vi "VAM-A-archive.vi"(1 "VAM-A":T2 {"63 B_NI6220" format="%.4g"; "62" format="%.4g"; "61" format="%.4g"; "60" format="%.4g"; "59" format="%.4g"; "58" format="%.4g"; "57" format="%.4g"; "56" format="%.4g"; "55" format="%.4g"; "54" format="%.4g"; "53" format="%.4g"; "52" format="%.4g"; "51" format="%.4g"; "50" format="%.4g"; "49" format="%.4g"; "48" format="%.4g"; "47" format="%.4g"; "46" format="%.4g"; "45" format="%.4g"; "44" format="%.4g"; "43" format="%.4g"; "42" format="%.4g"; "41" format="%.4g"; "40" format="%.4g"; "39 WCM2DMin" format="%.4g"; "38 WCM2GMin" format="%.4g"; "37 WCM2BMin" format="%.4g"; "36 WCM2HMin" format="%.4g"; "35 WCM2DMax" format="%.4g"; "34 WCM2GMax" format="%.4g"; "33 WCM2BMax" format="%.4g"; "32 WCM2HMax" format="%.4g"; "31" format="%.4g"; "30" format="%.4g"; "29" format="%.4g"; "28" format="%.4g"; "27" format="%.4g"; "26" format="%.4g"; "25" format="%.4g"; "24" format="%.4g"; "23" format="%.4g"; "22" format="%.4g"; "21" format="%.4g"; "20 ACQ Vide TPG300 PIQ63" format="%.4g"; "19 ACQ Libre" format="%.5g"; "18 ACQ Libre" format="%.5g"; "17 ACQ Vide Ecran PIQ53/63" format="%.5g"; "16 ACQ Vide Dip PIQ27/33" format="%.5g"; "15 ACQ Vide Miroir PIQ21" format="%.5g"; "14 ACQ Vide Section PIQ16" format="%.5g"; "13 ACQ Vide Canon PIQ12" format="%.5g"; "12 ACQ Vide PI Guide HF" format="%.5f"; "11 ACQ Vide Chambre" format="%.4g"; "10 ACQ Vide Section" format="%.4g"; "09" format="%.4g"; "08" format="%.4g"; "07" format="%.4g"; "06" format="%.4g"; "05" format="%.4g"; "04" format="%.4g"; "03" format="%.4g"; "02 ACQ Evénement" format="%.4g"; "01 ACQ Variables" format="%.4g"; "00 ACQ Auxiliare" format="%.4g"}, 2 "C5_IN_DIO96":T1, 3 "archive in":T3={"sync"={"elyse/sync/NI6071E/delay"=1.5500000000000005, "elyse/sync/NI6071E/width"=1.0, "elyse/sync/frequency/delay"=10.0, "elyse/sync/frequency/width"=181000.0, "elyse/sync/WCM/delay"=2177.9, "elyse/sync/WCM/width"=10.0, "elyse/sync/modulator/delay"=2182.400000000002, "elyse/sync/modulator/width"=3.0, "elyse/sync/HF/delay"=2175.0, "elyse/sync/HF/width"=3.0, "elyse/sync/Faraday/delay"=5080.0, "elyse/sync/Faraday/width"=100.0, "elyse/sync/Oscilloscope/delay"=2175.0, "elyse/sync/Oscilloscope/width"=2.8, "elyse/sync/50Hz_20MHz/delay"=1.0, "elyse/sync/50Hz_20MHz/width"=5000.0, "elyse/sync/laser_HF/delay"=0.35, "elyse/sync/laser_HF/width"=0.35, "elyse/sync/IMAC/delay"=2176.0, "elyse/sync/IMAC/width"=100.0, "elyse/sync/laser/delay"=2008.3, "elyse/sync/laser/width"=10.0, "elyse/sync/oscilloscope1/delay"=2175.0, "elyse/sync/oscilloscope1/width"=10.0, "elyse/sync/oscilloscope2/delay"=2175.0, "elyse/sync/oscilloscope2/width"=100.0, "elyse/sync/detection1/delay"=500.0, "elyse/sync/detection1/width"=500.0, "elyse/sync/detection1/delay"=0.3, "elyse/sync/detection2/width"=10.0, "elyse/sync/machine/delay"=2175.0, "elyse/sync/machine/width"=100.0, "elyse/sync/n_selection"=4.0}, "HT"={"elyse/HT/voltage/set_value"=6.5, "elyse/HT/voltage/value"=1.5625e-08, "elyse/HT/current/value"=0.0, "elyse/preamplifier/set_value"=1.5625e-08, "elyse/preamplifier/value"=0.0}, "HF"={"elyse/HF/attenuator/value"=-0.01903046052094623, "elyse/HF/dephaser/value"=-18.585806237727724, "elyse/HF/dephaser/value_manuel"=-78.82860725035081, "elyse/HF/canon/value"=0.0, "elyse/HF/section/value"=-18.585806237727724}, "vacuum"={"elyse/vacuum/preparation_chamber/state"=TRUE, "elyse/vacuum/preparation_chamber/measurement"=0.0, "elyse/vacuum/HF/state"=TRUE, "elyse/vacuum/HF/measurement"=0.0, "elyse/vacuum/canon/state"=TRUE, "elyse/vacuum/canon/measurement"=0.0, "elyse/vacuum/section/state"=TRUE, "elyse/vacuum/section/measurement"=0.0, "elyse/vacuum/dipole1/state"=TRUE, "elyse/vacuum/dipole1/measurement"=0.0, "elyse/vacuum/screen1/state"=TRUE, "elyse/vacuum/screen1/measurement"=0.0, "elyse/vacuum/mirror/state"=TRUE, "elyse/vacuum/mirror/measurement"=0.0, "elyse/vacuum/tpg300_section/state"=TRUE, "elyse/vacuum/tpg300_section/measurement"=0.0, "elyse/vacuum/valves/cathode/state"=FALSE, "elyse/vacuum/valves/injection/state"=FALSE}, "modulator"={"elyse/modulator/focale1/current/value"=0.0, "elyse/modulator/focale2/current/value"=0.0, "elyse/modulator/focale3/current/value"=0.0, "elyse/modulator/LAR/voltage/value"=0.0, "elyse/modulator/line_end/current/value"=0.0, "elyse/modulator/thyratron/currents/power/value"=0.0, "elyse/modulator/thyratron_reservoir/current/value"=0.0, "elyse/modulator/paramagnetization/current/value"=0.0, "elyse/modulator/thyratron/voltages/heating/value"=0.0, "elyse/modulator/thyratron/currents/heating/value"=0.0, "elyse/modulator/klystron/currents/power/value"=0.0, "elyse/modulator/klystron/voltages/power/value"=0.0, "elyse/modulator/klystron/currents/heating/value"=0.0, "elyse/modulator/klystron/voltages/heating/value"=0.0}, "cooling"={"elyse/cooling/section/temperature/set_value"=28.0, "elyse/cooling/section/temperature/measurement"=27.96142578125, "elyse/cooling/canon/temperature/set_value"=20.2, "elyse/cooling/canon/temperature/measurement"=26.69921875}, "magnets"={"elyse/magnets/focale/set_value"=0.0, "elyse/magnets/focale/value"=0.0, "elyse/magnets/phase_HF_laser/set_value"=0.0, "elyse/magnets/phase_HF_laser/value"=0.0, "elyse/magnets/dipole1/set_value"=0.0, "elyse/magnets/dipole1/value"=0.0, "elyse/magnets/dipole2/set_value"=0.0, "elyse/magnets/dipole2/value"=0.0, "elyse/magnets/Cor_H1/set_value"=0.0, "elyse/magnets/Cor_H1/value"=0.0, "elyse/magnets/Cor_V1/set_value"=0.0, "elyse/magnets/Cor_V1/value"=0.0, "elyse/magnets/Cor_H2/set_value"=0.0, "elyse/magnets/Cor_H2/value"=0.0, "elyse/magnets/Cor_V2/set_value"=0.0, "elyse/magnets/Cor_V2/value"=0.0, "elyse/magnets/Cor_H3/set_value"=0.0, "elyse/magnets/Cor_H3/value"=0.0, "elyse/magnets/Cor_V3/set_value"=-5.0, "elyse/magnets/Cor_V3/value"=0.0, "elyse/magnets/Cor_H4/set_value"=0.0, "elyse/magnets/Cor_H4/value"=0.0, "elyse/magnets/Cor_V4/set_value"=0.0, "elyse/magnets/Cor_V4/value"=0.0, "elyse/magnets/Cor_H5/set_value"=0.0, "elyse/magnets/Cor_H5/value"=0.0, "elyse/magnets/Cor_V5/set_value"=0.0, "elyse/magnets/Cor_V5/value"=0.0, "elyse/magnets/triplet1-1/set_value"=0.0, "elyse/magnets/triplet1-1/value"=0.0, "elyse/magnets/triplet1-2/set_value"=0.0, "elyse/magnets/triplet1-2/value"=0.0, "elyse/magnets/triplet2-1/set_value"=0.0, "elyse/magnets/triplet2-1/value"=0.0, "elyse/magnets/triplet2-2/set_value"=0.0, "elyse/magnets/triplet2-2/value"=0.0, "elyse/magnets/qudrupole1/set_value"=0.0, "elyse/magnets/qudrupole1/value"=0.0, "elyse/magnets/qudrupole2/set_value"=0.0, "elyse/magnets/qudrupole2/value"=0.0}, "time"={"elyse/timestamp"=0.0}}) -> (0 "archive out":T3={"sync"={"elyse/sync/NI6071E/delay"=1.5500000000000005, "elyse/sync/NI6071E/width"=1.0, "elyse/sync/frequency/delay"=10.0, "elyse/sync/frequency/width"=181000.0, "elyse/sync/WCM/delay"=2177.9, "elyse/sync/WCM/width"=10.0, "elyse/sync/modulator/delay"=2182.400000000002, "elyse/sync/modulator/width"=3.0, "elyse/sync/HF/delay"=2175.0, "elyse/sync/HF/width"=3.0, "elyse/sync/Faraday/delay"=5080.0, "elyse/sync/Faraday/width"=100.0, "elyse/sync/Oscilloscope/delay"=2175.0, "elyse/sync/Oscilloscope/width"=2.8, "elyse/sync/50Hz_20MHz/delay"=1.0, "elyse/sync/50Hz_20MHz/width"=5000.0, "elyse/sync/laser_HF/delay"=0.35, "elyse/sync/laser_HF/width"=0.35, "elyse/sync/IMAC/delay"=2176.0, "elyse/sync/IMAC/width"=100.0, "elyse/sync/laser/delay"=2008.3, "elyse/sync/laser/width"=10.0, "elyse/sync/oscilloscope1/delay"=2175.0, "elyse/sync/oscilloscope1/width"=10.0, "elyse/sync/oscilloscope2/delay"=2175.0, "elyse/sync/oscilloscope2/width"=100.0, "elyse/sync/detection1/delay"=500.0, "elyse/sync/detection1/width"=500.0, "elyse/sync/detection1/delay"=0.3, "elyse/sync/detection2/width"=10.0, "elyse/sync/machine/delay"=2175.0, "elyse/sync/machine/width"=100.0, "elyse/sync/n_selection"=4.0}, "HT"={"elyse/HT/voltage/set_value"=6.5, "elyse/HT/voltage/value"=1.5625e-08, "elyse/HT/current/value"=0.0, "elyse/preamplifier/set_value"=1.5625e-08, "elyse/preamplifier/value"=0.0}, "HF"={"elyse/HF/attenuator/value"=-0.01903046052094623, "elyse/HF/dephaser/value"=-18.585806237727724, "elyse/HF/dephaser/value_manuel"=-78.82860725035081, "elyse/HF/canon/value"=0.0, "elyse/HF/section/value"=-18.585806237727724}, "vacuum"={"elyse/vacuum/preparation_chamber/state"=TRUE, "elyse/vacuum/preparation_chamber/measurement"=0.0, "elyse/vacuum/HF/state"=TRUE, "elyse/vacuum/HF/measurement"=0.0, "elyse/vacuum/canon/state"=TRUE, "elyse/vacuum/canon/measurement"=0.0, "elyse/vacuum/section/state"=TRUE, "elyse/vacuum/section/measurement"=0.0, "elyse/vacuum/dipole1/state"=TRUE, "elyse/vacuum/dipole1/measurement"=0.0, "elyse/vacuum/screen1/state"=TRUE, "elyse/vacuum/screen1/measurement"=0.0, "elyse/vacuum/mirror/state"=TRUE, "elyse/vacuum/mirror/measurement"=0.0, "elyse/vacuum/tpg300_section/state"=TRUE, "elyse/vacuum/tpg300_section/measurement"=0.0, "elyse/vacuum/valves/cathode/state"=FALSE, "elyse/vacuum/valves/injection/state"=FALSE}, "modulator"={"elyse/modulator/focale1/current/value"=0.0, "elyse/modulator/focale2/current/value"=0.0, "elyse/modulator/focale3/current/value"=0.0, "elyse/modulator/LAR/voltage/value"=0.0, "elyse/modulator/line_end/current/value"=0.0, "elyse/modulator/thyratron/currents/power/value"=0.0, "elyse/modulator/thyratron_reservoir/current/value"=0.0, "elyse/modulator/paramagnetization/current/value"=0.0, "elyse/modulator/thyratron/voltages/heating/value"=0.0, "elyse/modulator/thyratron/currents/heating/value"=0.0, "elyse/modulator/klystron/currents/power/value"=0.0, "elyse/modulator/klystron/voltages/power/value"=0.0, "elyse/modulator/klystron/currents/heating/value"=0.0, "elyse/modulator/klystron/voltages/heating/value"=0.0}, "cooling"={"elyse/cooling/section/temperature/set_value"=28.0, "elyse/cooling/section/temperature/measurement"=27.96142578125, "elyse/cooling/canon/temperature/set_value"=20.2, "elyse/cooling/canon/temperature/measurement"=26.69921875}, "magnets"={"elyse/magnets/focale/set_value"=0.0, "elyse/magnets/focale/value"=0.0, "elyse/magnets/phase_HF_laser/set_value"=0.0, "elyse/magnets/phase_HF_laser/value"=0.0, "elyse/magnets/dipole1/set_value"=0.0, "elyse/magnets/dipole1/value"=0.0, "elyse/magnets/dipole2/set_value"=0.0, "elyse/magnets/dipole2/value"=0.0, "elyse/magnets/Cor_H1/set_value"=0.0, "elyse/magnets/Cor_H1/value"=0.0, "elyse/magnets/Cor_V1/set_value"=0.0, "elyse/magnets/Cor_V1/value"=0.0, "elyse/magnets/Cor_H2/set_value"=0.0, "elyse/magnets/Cor_H2/value"=0.0, "elyse/magnets/Cor_V2/set_value"=0.0, "elyse/magnets/Cor_V2/value"=0.0, "elyse/magnets/Cor_H3/set_value"=0.0, "elyse/magnets/Cor_H3/value"=0.0, "elyse/magnets/Cor_V3/set_value"=-5.0, "elyse/magnets/Cor_V3/value"=0.0, "elyse/magnets/Cor_H4/set_value"=0.0, "elyse/magnets/Cor_H4/value"=0.0, "elyse/magnets/Cor_V4/set_value"=0.0, "elyse/magnets/Cor_V4/value"=0.0, "elyse/magnets/Cor_H5/set_value"=0.0, "elyse/magnets/Cor_H5/value"=0.0, "elyse/magnets/Cor_V5/set_value"=0.0, "elyse/magnets/Cor_V5/value"=0.0, "elyse/magnets/triplet1-1/set_value"=0.0, "elyse/magnets/triplet1-1/value"=0.0, "elyse/magnets/triplet1-2/set_value"=0.0, "elyse/magnets/triplet1-2/value"=0.0, "elyse/magnets/triplet2-1/set_value"=0.0, "elyse/magnets/triplet2-1/value"=0.0, "elyse/magnets/triplet2-2/set_value"=0.0, "elyse/magnets/triplet2-2/value"=0.0, "elyse/magnets/qudrupole1/set_value"=0.0, "elyse/magnets/qudrupole1/value"=0.0, "elyse/magnets/qudrupole2/set_value"=0.0, "elyse/magnets/qudrupole2/value"=0.0}, "time"={"elyse/timestamp"=0.0}})   [LabVIEW 2020]
uses:
  archive.ctl
  sync_type_def.ctl
  HT_type-def.ctl
  HF_type_def.ctl
  vacuum_type_def.ctl
  modulator_type_def.ctl
  water_cooling_type_def.ctl
  all_magnets_type_def.ctl
  <vilib>/ptbypt/NI_PtbyPt.lvlib
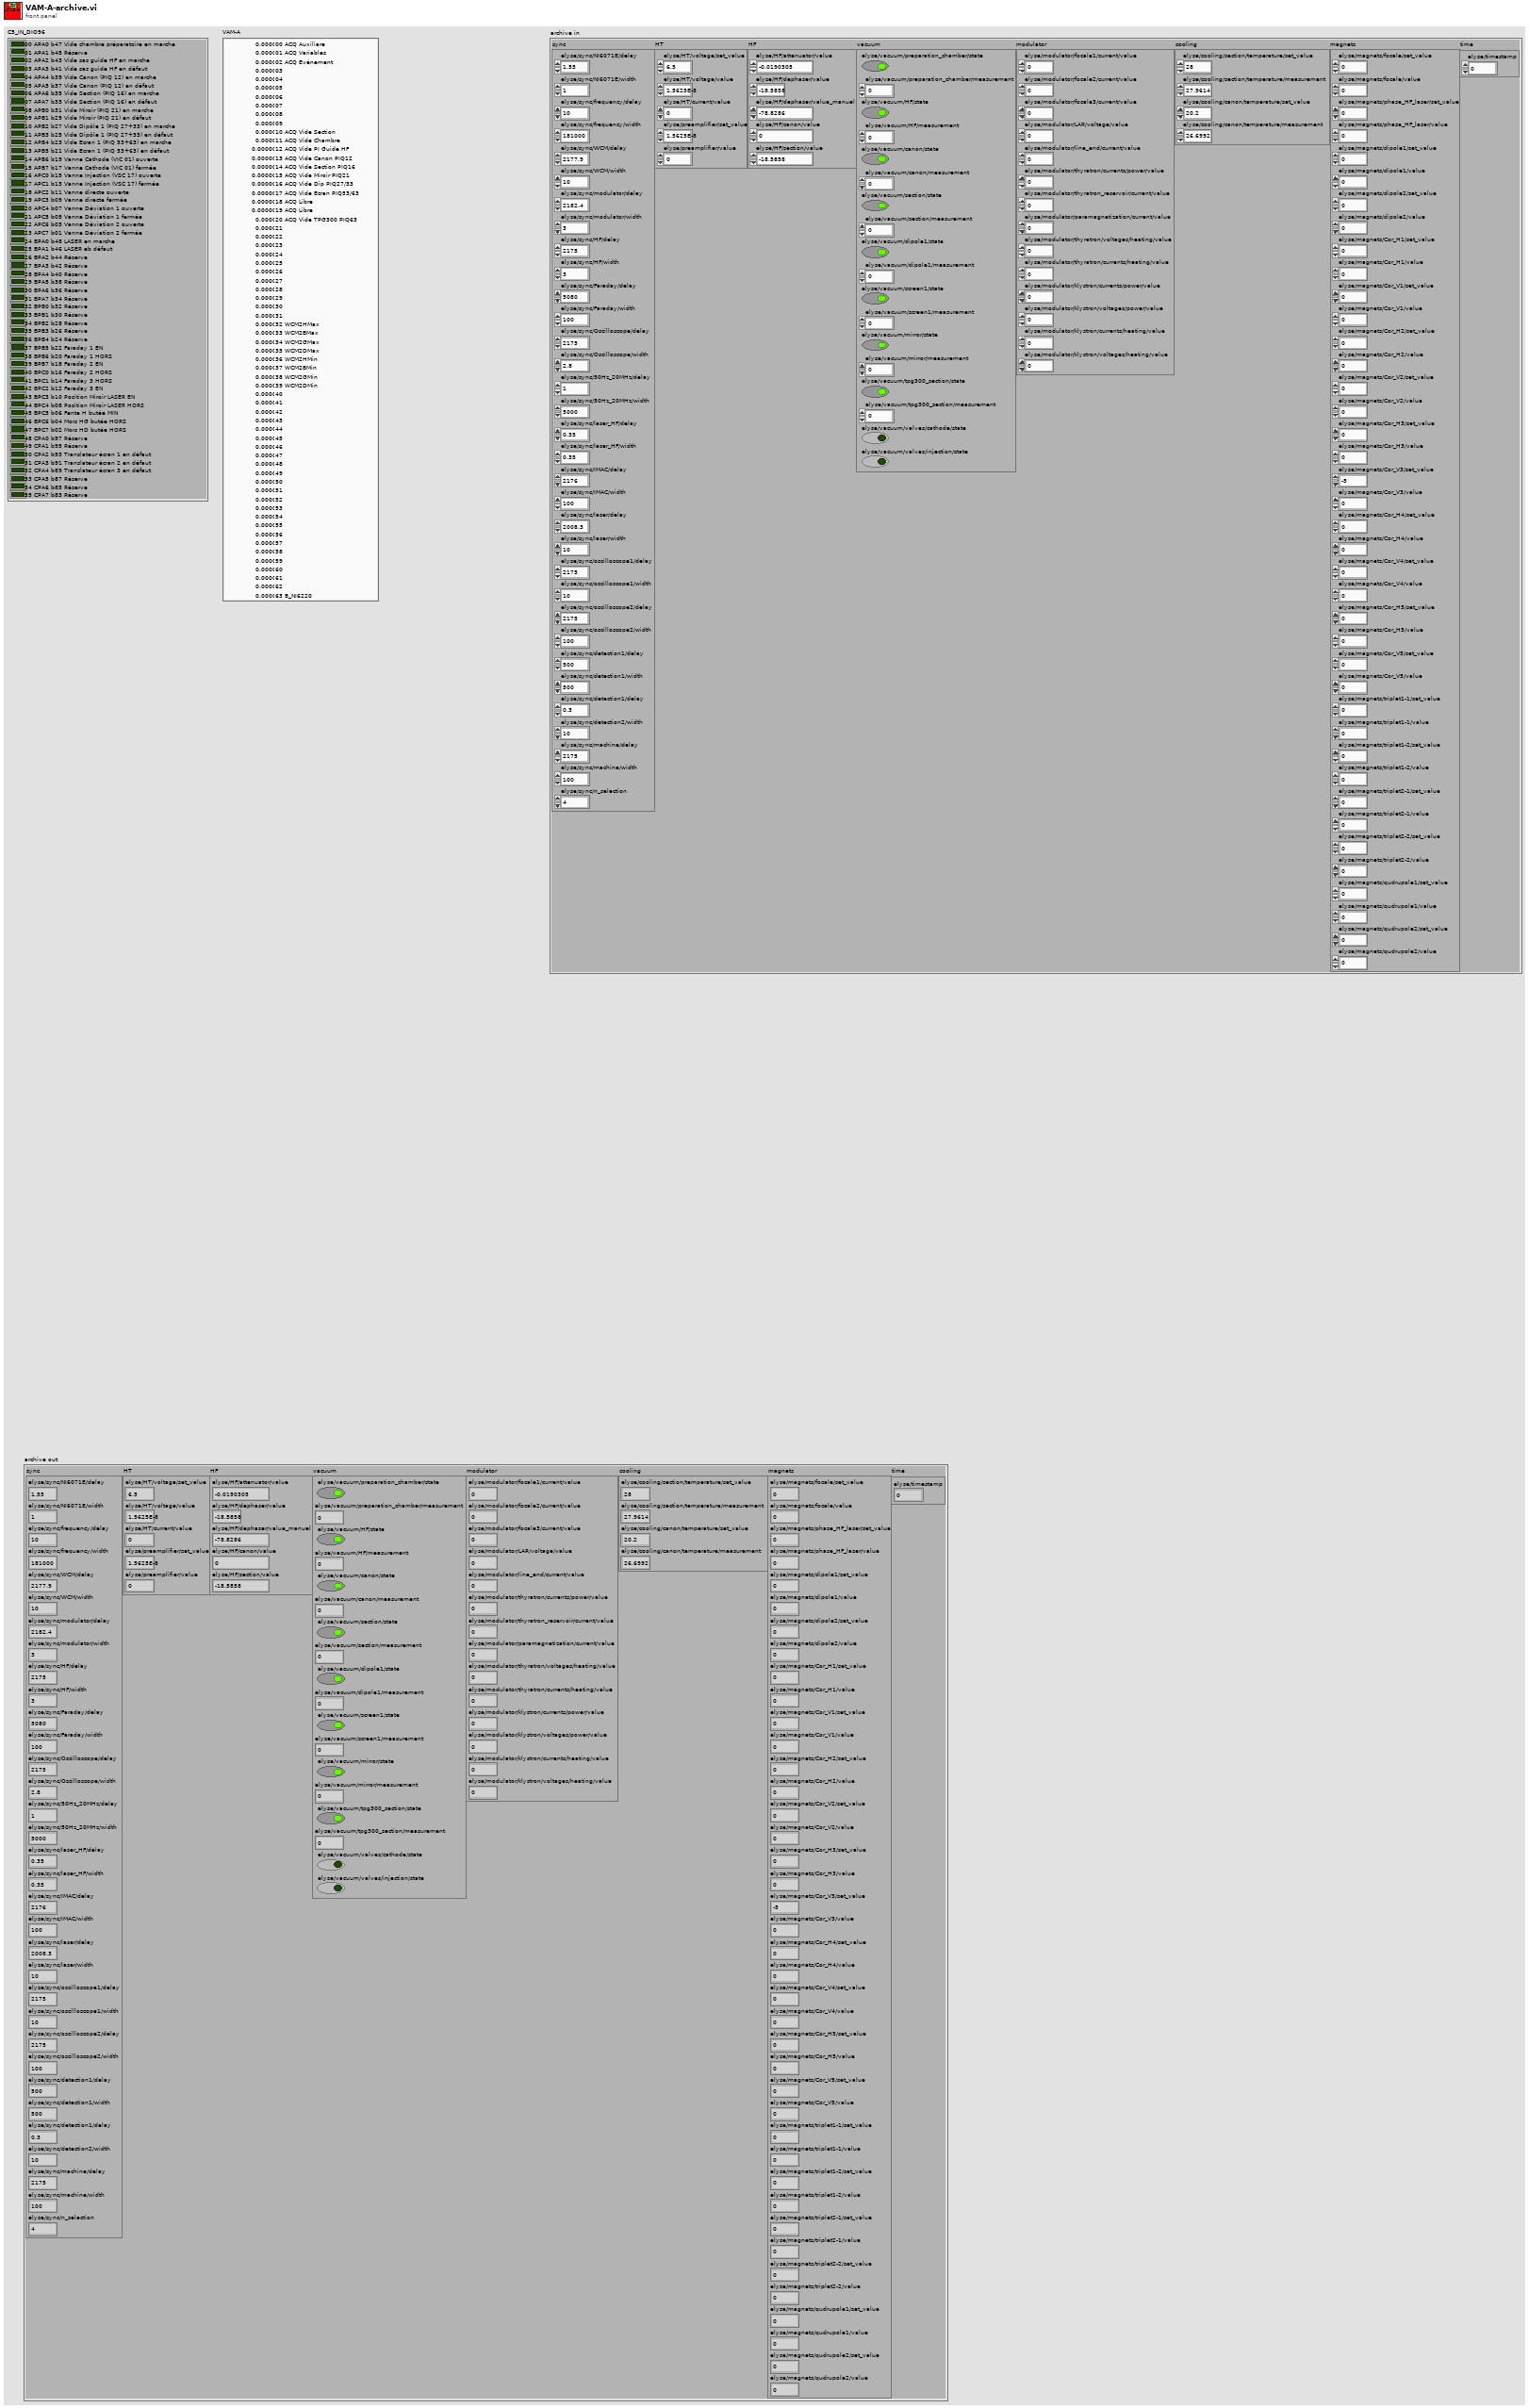
[diagram p1: front panel]
types:
  T1 = cluster{"00 APA0 b47 Vide chambre préparatoire en marche":bool, "01 APA1 b45 Réserve":bool, "02 APA2 b43 Vide sas guide HF en marche":bool, "03 APA3 b41 Vide sas guide HF en défaut":bool, "04 APA4 b39 Vide Canon (PIQ 12) en marche":bool, "05 APA5 b37 Vide Canon (PIQ 12) en défaut":bool, "06 APA6 b35 Vide Section (PIQ 16) en marche":bool, "07 APA7 b33 Vide Section (PIQ 16) en défaut":bool, "08 APB0 b31 Vide Miroir (PIQ 21) en marche":bool, "09 APB1 b29 Vide Miroir (PIQ 21) en défaut":bool, "10 APB2 b27 Vide Dipôle 1 (PIQ 27+33) en marche":bool, "11 APB3 b25 Vide Dipôle 1 (PIQ 27+33) en défaut":bool, "12 APB4 b23 Vide Ecran 1 (PIQ 53+63) en marche":bool, "13 APB5 b21 Vide Ecran 1 (PIQ 53+63) en défaut":bool, "14 APB6 b19 Vanne Cathode (VIC 01) ouverte":bool, "15 APB7 b17 Vanne Cathode (VIC 01) fermée":bool, "16 APC0 b15 Vanne Injection (VSC 17) ouverte":bool, "17 APC1 b13 Vanne Injection (VSC 17) fermée":bool, "18 APC2 b11 Vanne directe ouverte":bool, "19 APC3 b09 Vanne directe fermée":bool, "20 APC4 b07 Vanne Déviation 1 ouverte":bool, "21 APC5 b05 Vanne Déviation 1 fermée":bool, "22 APC6 b03 Vanne Déviation 2 ouverte":bool, "23 APC7 b01 Vanne Déviation 2 fermée":bool, "24 BPA0 b48 LASER en marche":bool, "25 BPA1 b46 LASER eb défaut":bool, "26 BPA2 b44 Réserve":bool, "27 BPA3 b42 Réserve":bool, "28 BPA4 b40 Réserve":bool, "29 BPA5 b38 Réserve":bool, "30 BPA6 b36 Réserve":bool, "31 BPA7 b34 Réserve":bool, "32 BPB0 b32 Réserve":bool, "33 BPB1 b30 Réserve":bool, "34 BPB2 b28 Réserve":bool, "35 BPB3 b26 Réserve":bool, "36 BPB4 b24 Réserve":bool, "37 BPB5 b22 Faraday 1 EN":bool, "38 BPB6 b20 Faraday 1 HORS":bool, "39 BPB7 b18 Faraday 2 EN":bool, "40 BPC0 b16 Faraday 2 HORS":bool, "41 BPC1 b14 Faraday 3 HORS":bool, "42 BPC2 b12 Faraday 3 EN":bool, "43 BPC3 b10 Position Miroir LASER EN":bool, "44 BPC4 b08 Position Miroir LASER HORS":bool, "45 BPC5 b06 Fente H butée MIN":bool, "46 BPC6 b04 Mors HG butée HORS":bool, "47 BPC7 b02 Mors HD butée HORS":bool, "48 CPA0 b97 Réserve":bool, "49 CPA1 b95 Réserve":bool, "50 CPA2 b93 Translateur écran 1 en défaut":bool, "51 CPA3 b91 Translateur écran 2 en défaut":bool, "52 CPA4 b89 Translateur écran 3 en défaut":bool, "53 CPA5 b87 Réserve":bool, "54 CPA6 b85 Réserve":bool, "55 CPA7 b83 Réserve":bool}
  T2 = cluster{"00 ACQ Auxiliare":dbl, "01 ACQ Variables":dbl, "02 ACQ Evénement":dbl, "03 ":dbl, "04":dbl, "05":dbl, "06":dbl, "07":dbl, "08":dbl, "09":dbl, "10 ACQ Vide Section":dbl, "11 ACQ Vide Chambre":dbl, "12 ACQ Vide PI Guide HF":dbl, "13 ACQ Vide Canon PIQ12":dbl, "14 ACQ Vide Section PIQ16":dbl, "15 ACQ Vide Miroir PIQ21":dbl, "16 ACQ Vide Dip PIQ27/33 ":dbl, "17 ACQ Vide Ecran PIQ53/63":dbl, "18 ACQ Libre":dbl, "19 ACQ Libre":dbl, "20 ACQ Vide TPG300 PIQ63":dbl, "21":dbl, "22":dbl, "23":dbl, "24":dbl, "25":dbl, "26":dbl, "27":dbl, "28":dbl, "29":dbl, "30":dbl, "31":dbl, "32 WCM2HMax":dbl, "33 WCM2BMax":dbl, "34 WCM2GMax":dbl, "35 WCM2DMax":dbl, "36 WCM2HMin":dbl, "37 WCM2BMin":dbl, "38 WCM2GMin":dbl, "39 WCM2DMin":dbl, "40":dbl, "41":dbl, "42":dbl, "43":dbl, "44":dbl, "45":dbl, "46":dbl, "47":dbl, "48":dbl, "49":dbl, "50":dbl, "51":dbl, "52":dbl, "53":dbl, "54":dbl, "55":dbl, "56":dbl, "57":dbl, "58":dbl, "59":dbl, "60":dbl, "61":dbl, "62":dbl, "63 B_NI6220":dbl}
  T3 = typedef "archive.ctl" = cluster{"sync":T4, "HT":T5, "HF":T6, "vacuum":T7, "modulator":T8, "cooling":T9, "magnets":T10, "time":cluster{"elyse/timestamp":dbl}}
  T4 = typedef "sync_type_def.ctl" = cluster{"elyse/sync/NI6071E/delay":dbl, "elyse/sync/NI6071E/width":dbl, "elyse/sync/frequency/delay":dbl, "elyse/sync/frequency/width":dbl, "elyse/sync/WCM/delay":dbl, "elyse/sync/WCM/width":dbl, "elyse/sync/modulator/delay":dbl, "elyse/sync/modulator/width":dbl, "elyse/sync/HF/delay":dbl, "elyse/sync/HF/width":dbl, "elyse/sync/Faraday/delay":dbl, "elyse/sync/Faraday/width":dbl, "elyse/sync/Oscilloscope/delay":dbl, "elyse/sync/Oscilloscope/width":dbl, "elyse/sync/50Hz_20MHz/delay":dbl, "elyse/sync/50Hz_20MHz/width":dbl, "elyse/sync/laser_HF/delay":dbl, "elyse/sync/laser_HF/width":dbl, "elyse/sync/IMAC/delay":dbl, "elyse/sync/IMAC/width":dbl, "elyse/sync/laser/delay":dbl, "elyse/sync/laser/width":dbl, "elyse/sync/oscilloscope1/delay":dbl, "elyse/sync/oscilloscope1/width":dbl, "elyse/sync/oscilloscope2/delay":dbl, "elyse/sync/oscilloscope2/width":dbl, "elyse/sync/detection1/delay":dbl, "elyse/sync/detection1/width":dbl, "elyse/sync/detection1/delay":dbl, "elyse/sync/detection2/width":dbl, "elyse/sync/machine/delay":dbl, "elyse/sync/machine/width":dbl, "elyse/sync/n_selection":dbl}
  T5 = typedef "HT_type-def.ctl" = cluster{"elyse/HT/voltage/set_value":dbl, "elyse/HT/voltage/value":dbl, "elyse/HT/current/value":dbl, "elyse/preamplifier/set_value":dbl, "elyse/preamplifier/value":dbl}
  T6 = typedef "HF_type_def.ctl" = cluster{"elyse/HF/attenuator/value":dbl, "elyse/HF/dephaser/value":dbl, "elyse/HF/dephaser/value_manuel":dbl, "elyse/HF/canon/value":dbl, "elyse/HF/section/value":dbl}
  T7 = typedef "vacuum_type_def.ctl" = cluster{"elyse/vacuum/preparation_chamber/state":bool, "elyse/vacuum/preparation_chamber/measurement":dbl, "elyse/vacuum/HF/state":bool, "elyse/vacuum/HF/measurement":dbl, "elyse/vacuum/canon/state":bool, "elyse/vacuum/canon/measurement":dbl, "elyse/vacuum/section/state":bool, "elyse/vacuum/section/measurement":dbl, "elyse/vacuum/dipole1/state":bool, "elyse/vacuum/dipole1/measurement":dbl, "elyse/vacuum/screen1/state":bool, "elyse/vacuum/screen1/measurement":dbl, "elyse/vacuum/mirror/state":bool, "elyse/vacuum/mirror/measurement":dbl, "elyse/vacuum/tpg300_section/state":bool, "elyse/vacuum/tpg300_section/measurement":dbl, "elyse/vacuum/valves/cathode/state":bool, "elyse/vacuum/valves/injection/state":bool}
  T8 = typedef "modulator_type_def.ctl" = cluster{"elyse/modulator/focale1/current/value":dbl, "elyse/modulator/focale2/current/value":dbl, "elyse/modulator/focale3/current/value":dbl, "elyse/modulator/LAR/voltage/value":dbl, "elyse/modulator/line_end/current/value":dbl, "elyse/modulator/thyratron/currents/power/value":dbl, "elyse/modulator/thyratron_reservoir/current/value":dbl, "elyse/modulator/paramagnetization/current/value":dbl, "elyse/modulator/thyratron/voltages/heating/value":dbl, "elyse/modulator/thyratron/currents/heating/value":dbl, "elyse/modulator/klystron/currents/power/value":dbl, "elyse/modulator/klystron/voltages/power/value":dbl, "elyse/modulator/klystron/currents/heating/value":dbl, "elyse/modulator/klystron/voltages/heating/value":dbl}
  T9 = typedef "water_cooling_type_def.ctl" = cluster{"elyse/cooling/section/temperature/set_value":dbl, "elyse/cooling/section/temperature/measurement":dbl, "elyse/cooling/canon/temperature/set_value":dbl, "elyse/cooling/canon/temperature/measurement":dbl}
  T10 = typedef "all_magnets_type_def.ctl" = cluster{"elyse/magnets/focale/set_value":dbl, "elyse/magnets/focale/value":dbl, "elyse/magnets/phase_HF_laser/set_value":dbl, "elyse/magnets/phase_HF_laser/value":dbl, "elyse/magnets/dipole1/set_value":dbl, "elyse/magnets/dipole1/value":dbl, "elyse/magnets/dipole2/set_value":dbl, "elyse/magnets/dipole2/value":dbl, "elyse/magnets/Cor_H1/set_value":dbl, "elyse/magnets/Cor_H1/value":dbl, "elyse/magnets/Cor_V1/set_value":dbl, "elyse/magnets/Cor_V1/value":dbl, "elyse/magnets/Cor_H2/set_value":dbl, "elyse/magnets/Cor_H2/value":dbl, "elyse/magnets/Cor_V2/set_value":dbl, "elyse/magnets/Cor_V2/value":dbl, "elyse/magnets/Cor_H3/set_value":dbl, "elyse/magnets/Cor_H3/value":dbl, "elyse/magnets/Cor_V3/set_value":dbl, "elyse/magnets/Cor_V3/value":dbl, "elyse/magnets/Cor_H4/set_value":dbl, "elyse/magnets/Cor_H4/value":dbl, "elyse/magnets/Cor_V4/set_value":dbl, "elyse/magnets/Cor_V4/value":dbl, "elyse/magnets/Cor_H5/set_value":dbl, "elyse/magnets/Cor_H5/value":dbl, "elyse/magnets/Cor_V5/set_value":dbl, "elyse/magnets/Cor_V5/value":dbl, "elyse/magnets/triplet1-1/set_value":dbl, "elyse/magnets/triplet1-1/value":dbl, "elyse/magnets/triplet1-2/set_value":dbl, "elyse/magnets/triplet1-2/value":dbl, "elyse/magnets/triplet2-1/set_value":dbl, "elyse/magnets/triplet2-1/value":dbl, "elyse/magnets/triplet2-2/set_value":dbl, "elyse/magnets/triplet2-2/value":dbl, "elyse/magnets/qudrupole1/set_value":dbl, "elyse/magnets/qudrupole1/value":dbl, "elyse/magnets/qudrupole2/set_value":dbl, "elyse/magnets/qudrupole2/value":dbl}
  T11 = cluster{"[0]":dbl, "[1]":dbl, "[2]":dbl, "[3]":dbl, "[4]":dbl, "[5]":dbl}
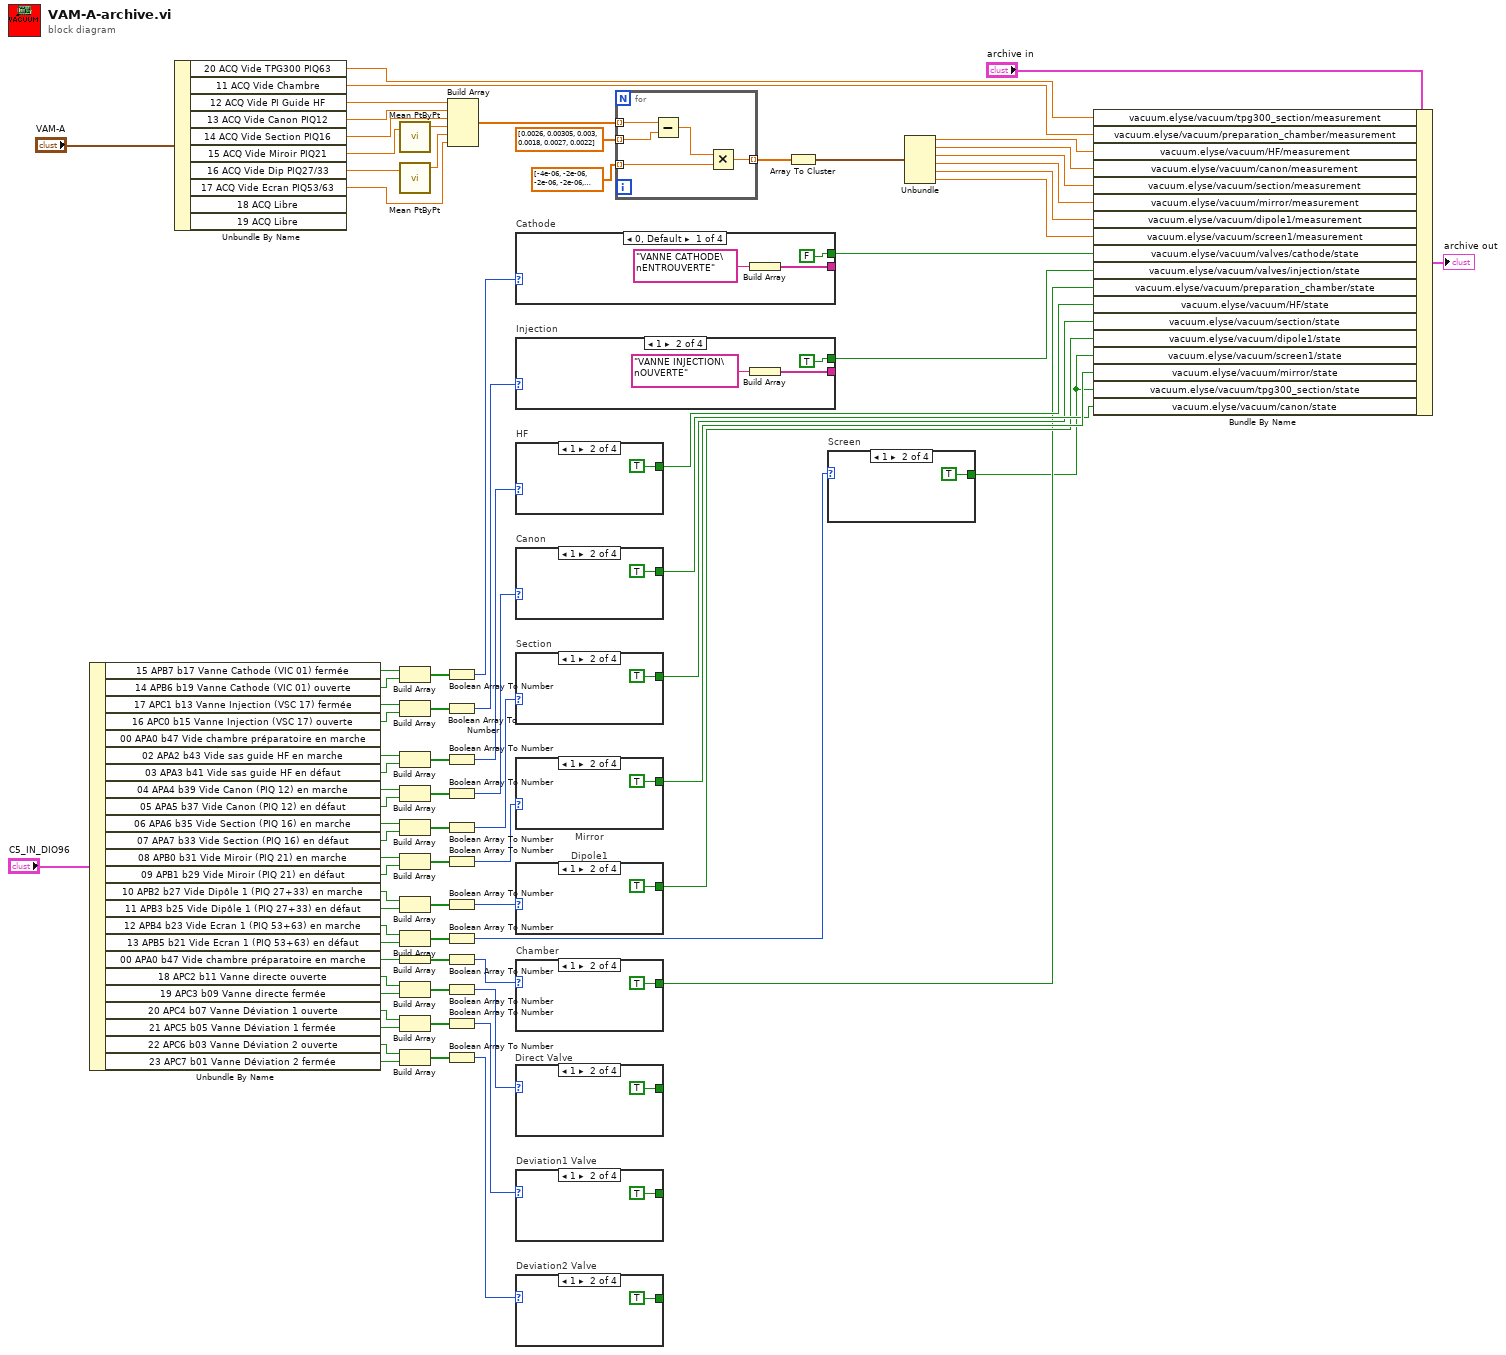
[diagram p0: block diagram]
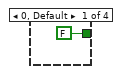
[diagram p2: hidden frame]
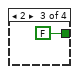
[diagram p3: hidden frame]
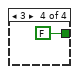
[diagram p4: hidden frame]
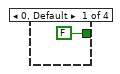
[diagram p5: hidden frame]
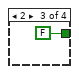
[diagram p6: hidden frame]
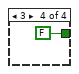
[diagram p7: hidden frame]
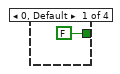
[diagram p8: hidden frame]
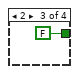
[diagram p9: hidden frame]
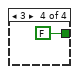
[diagram p10: hidden frame]
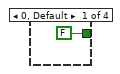
[diagram p11: hidden frame]
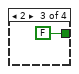
[diagram p12: hidden frame]
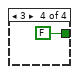
[diagram p13: hidden frame]
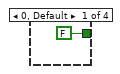
[diagram p14: hidden frame]
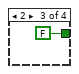
[diagram p15: hidden frame]
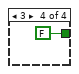
[diagram p16: hidden frame]
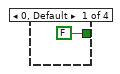
[diagram p17: hidden frame]
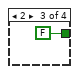
[diagram p18: hidden frame]
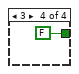
[diagram p19: hidden frame]
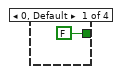
[diagram p20: hidden frame]
diagram:
  n1 = Unbundle By Name("C5_IN_DIO96") -> ("15 APB7 b17 Vanne Cathode (VIC 01) fermée"=w56:bool, "14 APB6 b19 Vanne Cathode (VIC 01) ouverte"=w55:bool, "17 APC1 b13 Vanne Injection (VSC 17) fermée"=w49:bool, "16 APC0 b15 Vanne Injection (VSC 17) ouverte"=w48:bool, "02 APA2 b43 Vide sas guide HF en marche"=w30:bool, "03 APA3 b41 Vide sas guide HF en défaut"=w29:bool, "04 APA4 b39 Vide Canon (PIQ 12) en marche"=w46:bool, "05 APA5 b37 Vide Canon (PIQ 12) en défaut"=w45:bool, "06 APA6 b35 Vide Section (PIQ 16) en marche"=w35:bool, "07 APA7 b33 Vide Section (PIQ 16) en défaut"=w34:bool, "08 APB0 b31 Vide Miroir (PIQ 21) en marche"=w41:bool, "09 APB1 b29 Vide Miroir (PIQ 21) en défaut"=w40:bool, "10 APB2 b27 Vide Dipôle 1 (PIQ 27+33) en marche"=w21:bool, "11 APB3 b25 Vide Dipôle 1 (PIQ 27+33) en défaut"=w22:bool, "12 APB4 b23 Vide Ecran 1 (PIQ 53+63) en marche"=w25:bool, "13 APB5 b21 Vide Ecran 1 (PIQ 53+63) en défaut"=w24:bool, "00 APA0 b47 Vide chambre préparatoire en marche"=w17:bool, "18 APC2 b11 Vanne directe ouverte"=w8:bool, "19 APC3 b09 Vanne directe fermée"=w7:bool, "20 APC4 b07 Vanne Déviation 1 ouverte"=w13:bool, "21 APC5 b05 Vanne Déviation 1 fermée"=w12:bool, "22 APC6 b03 Vanne Déviation 2 ouverte"=w11:bool, "23 APC7 b01 Vanne Déviation 2 fermée"=w10:bool)  [unwired: 1 out]
  n2 = Unbundle By Name("VAM-A") -> ("20 ACQ Vide TPG300 PIQ63"=w81:dbl, "11 ACQ Vide Chambre"=w80:dbl, "12 ACQ Vide PI Guide HF"=w66:dbl, "13 ACQ Vide Canon PIQ12"=w65:dbl, "14 ACQ Vide Section PIQ16"=w64:dbl, "15 ACQ Vide Miroir PIQ21"=w63:dbl, "16 ACQ Vide Dip PIQ27/33"=w62:dbl, "17 ACQ Vide Ecran PIQ53/63"=w61:dbl)  [unwired: 2 out]
  n3 = call <vilib>:"Mean PtByPt.vi"("x"=w63) -> ("mean"=w72:dbl)  [unwired: 3 in, 1 out]
  n4 = call <vilib>:"Mean PtByPt.vi"("x"=w62) -> ("mean"=w73:dbl)  [unwired: 3 in, 1 out]
  n5 = Build Array(w56, w55) -> (w57:bool[])
  n6 = Build Array(w49, w48) -> (w53:bool[])
  n7 = Build Array(w30, w29) -> (w31:bool[])
  n8 = Build Array(w46, w45) -> (w47:bool[])
  n9 = Build Array(w35, w34) -> (w37:bool[])
  n10 = Build Array(w41, w40) -> (w43:bool[])
  n11 = Build Array(w21, w22) -> (w23:bool[])
  n12 = Build Array(w25, w24) -> (w27:bool[])
  n13 = Build Array(w17) -> (w18:bool[])
  n14 = Build Array(w8, w7) -> (w9:bool[])
  n15 = Build Array(w13, w12) -> (w14:bool[])
  n16 = Build Array(w11, w10) -> (w3:bool[])
  n17 = Boolean Array To Number(Boolean array=w57) -> (number=w54:u32)
  n18 = Boolean Array To Number(Boolean array=w53) -> (number=w52:u32)
  n19 = Boolean Array To Number(Boolean array=w31) -> (number=w28:u32)
  n20 = Boolean Array To Number(Boolean array=w47) -> (number=w44:u32)
  n21 = Boolean Array To Number(Boolean array=w37) -> (number=w36:u32)
  n22 = Boolean Array To Number(Boolean array=w43) -> (number=w42:u32)
  n23 = Boolean Array To Number(Boolean array=w23) -> (number=w20:u32)
  n24 = Boolean Array To Number(Boolean array=w27) -> (number=w26:u32)
  n25 = Boolean Array To Number(Boolean array=w18) -> (number=w16:u32)
  n26 = Boolean Array To Number(Boolean array=w9) -> (number=w6:u32)
  n27 = Boolean Array To Number(Boolean array=w14) -> (number=w5:u32)
  n28 = Boolean Array To Number(Boolean array=w3) -> (number=w4:u32)
  n29 = Build Array(w66, w65, w64, w72, w73, w61) -> (w69:dbl[])
  n30 = case "Cathode" shown="0, Default" w54 {
    tunnel: [w83 w86 w89 w92] -> _
    tunnel: [FALSE TRUE FALSE FALSE] -> w51
    frame 0, Default {
      n31 = Build Array("VANNE CATHODE\nENTROUVERTE" ("source")) -> (w83:string[])
    }
    frame 1 {
      n32 = Build Array("VANNE CATHODE\nOUVERTE" ("source")) -> (w86:string[])
    }
    frame 2 {
      n33 = Build Array("VANNE CATHODE\nFERMEE" ("source")) -> (w89:string[])
    }
    frame 3 {
      n34 = Build Array("VANNE CATHODE\nEN DEFAUT" ("source")) -> (w92:string[])
    }
  }
  n35 = case "Injection" shown="1" w52 {
    tunnel: [w95 w98 w101 w104] -> _
    tunnel: [FALSE TRUE FALSE FALSE] -> w50
    frame 0, Default {
      n36 = Build Array("VANNE INJECTION\nENTROUVERTE" ("source")) -> (w95:string[])
    }
    frame 1 {
      n37 = Build Array("VANNE INJECTION\nOUVERTE" ("source")) -> (w98:string[])
    }
    frame 2 {
      n38 = Build Array("VANNE INJECTION\nFERMEE" ("source")) -> (w101:string[])
    }
    frame 3 {
      n39 = Build Array("VANNE INJECTION\nEN DEFAUT" ("source")) -> (w104:string[])
    }
  }
  n40 = case "HF" shown="1" w28 {
    tunnel: [FALSE TRUE FALSE FALSE] -> w32
    frame 0, Default {
    }
    frame 1 {
    }
    frame 2 {
    }
    frame 3 {
    }
  }
  n41 = case "Canon" shown="1" w44 {
    tunnel: [FALSE TRUE FALSE FALSE] -> w38
    frame 0, Default {
    }
    frame 1 {
    }
    frame 2 {
    }
    frame 3 {
    }
  }
  n42 = case "Section" shown="1" w36 {
    tunnel: [FALSE TRUE FALSE FALSE] -> w33
    frame 0, Default {
    }
    frame 1 {
    }
    frame 2 {
    }
    frame 3 {
    }
  }
  n43 = case "Mirror" shown="1" w42 {
    tunnel: [FALSE TRUE FALSE FALSE] -> w39
    frame 0, Default {
    }
    frame 1 {
    }
    frame 2 {
    }
    frame 3 {
    }
  }
  n44 = case "Dipole1" shown="1" w20 {
    tunnel: [FALSE TRUE FALSE FALSE] -> w19
    frame 0, Default {
    }
    frame 1 {
    }
    frame 2 {
    }
    frame 3 {
    }
  }
  n45 = case "Chamber" shown="1" w16 {
    tunnel: [FALSE TRUE FALSE FALSE] -> w15
    frame 0, Default {
    }
    frame 1 {
    }
    frame 2 {
    }
    frame 3 {
    }
  }
  n46 = case "Direct Valve" shown="1" w6 {
    tunnel: [FALSE TRUE FALSE FALSE] -> _
    frame 0, Default {
    }
    frame 1 {
    }
    frame 2 {
    }
    frame 3 {
    }
  }
  n47 = case "Deviation1 Valve" shown="1" w5 {
    tunnel: [FALSE TRUE FALSE FALSE] -> _
    frame 0, Default {
    }
    frame 1 {
    }
    frame 2 {
    }
    frame 3 {
    }
  }
  n48 = case "Deviation2 Valve" shown="1" w4 {
    tunnel: [FALSE TRUE FALSE FALSE] -> _
    frame 0, Default {
    }
    frame 1 {
    }
    frame 2 {
    }
    frame 3 {
    }
  }
  n49 = for {
    tunnel: dbl[] [-4e-06, -2e-06, -2e-06, -2e-06, -1e-06, -1e-06] -> [w143] mode=indexing
    tunnel: dbl[] [0.0026, 0.00305, 0.003, 0.0018, 0.0027, 0.0022] -> [w145] mode=indexing
    tunnel: w69 -> [w146] mode=indexing
    tunnel: [w142] -> w70 mode=indexing
    n50 = Subtract(x=w146, y=w145) -> (x-y=w144:dbl)
    n51 = Multiply(x=w144, y=w143) -> (x*y=w142:dbl)
  }
  n52 = Array To Cluster(array=w70) -> (cluster=w71:T11)
  n53 = case "Screen" shown="1" w26 {
    tunnel: [FALSE TRUE FALSE FALSE] -> w2
    frame 0, Default {
    }
    frame 1 {
    }
    frame 2 {
    }
    frame 3 {
    }
  }
  n54 = Unbundle(w71) -> ("[0]"=w79:dbl, "[1]"=w78:dbl, "[2]"=w76:dbl, "[3]"=w75:dbl, "[4]"=w74:dbl, "[5]"=w77:dbl)
  n55 = Bundle By Name(cluster="archive in", "vacuum.elyse/vacuum/tpg300_section/measurement"=w81, "vacuum.elyse/vacuum/preparation_chamber/measurement"=w80, "vacuum.elyse/vacuum/HF/measurement"=w79, "vacuum.elyse/vacuum/canon/measurement"=w78, "vacuum.elyse/vacuum/section/measurement"=w76, "vacuum.elyse/vacuum/mirror/measurement"=w75, "vacuum.elyse/vacuum/dipole1/measurement"=w74, "vacuum.elyse/vacuum/screen1/measurement"=w77, "vacuum.elyse/vacuum/valves/cathode/state"=w51, "vacuum.elyse/vacuum/valves/injection/state"=w50, "vacuum.elyse/vacuum/preparation_chamber/state"=w15, "vacuum.elyse/vacuum/HF/state"=w32, "vacuum.elyse/vacuum/section/state"=w33, "vacuum.elyse/vacuum/dipole1/state"=w19, "vacuum.elyse/vacuum/screen1/state"=w2, "vacuum.elyse/vacuum/mirror/state"=w39, "vacuum.elyse/vacuum/tpg300_section/state"=w2, "vacuum.elyse/vacuum/canon/state"=w38) -> (→"archive out":T3)
